vi "read single param.vi"(8 "error in (no error)":errorcluster, 10 "Parameter":string, 11 "PSP-603 in":refnum<class "PSP-603.lvclass">) -> (0 "error out":errorcluster, 2 "Data":string, 3 "PSP-603 out":refnum<class "PSP-603.lvclass">)   [LabVIEW 2025, in "Power Supply.lvlib" / "PSP-603.lvclass"]
uses:
  PSP-603.lvclass
  PSP-603.lvclass/PSP-603.ctl
panel:
  out "concatenated string":string
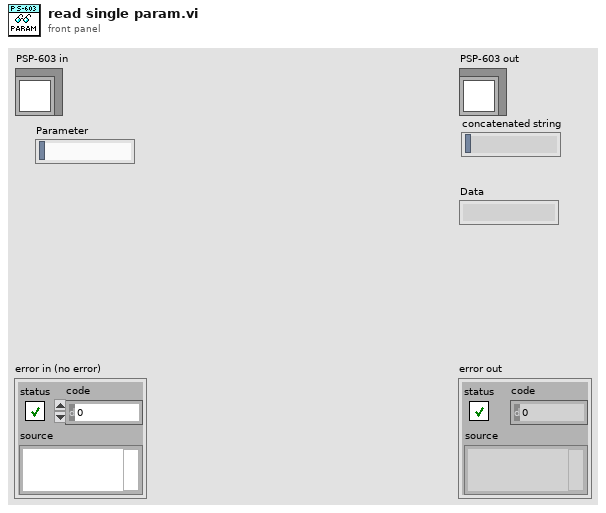
[diagram p1: front panel]
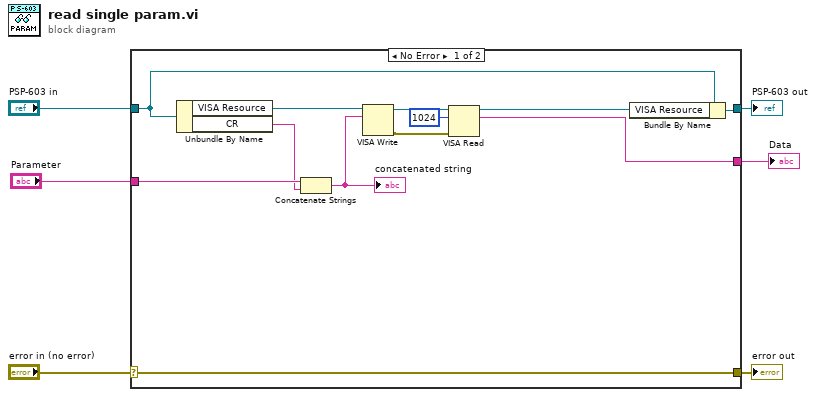
[diagram p0: block diagram]
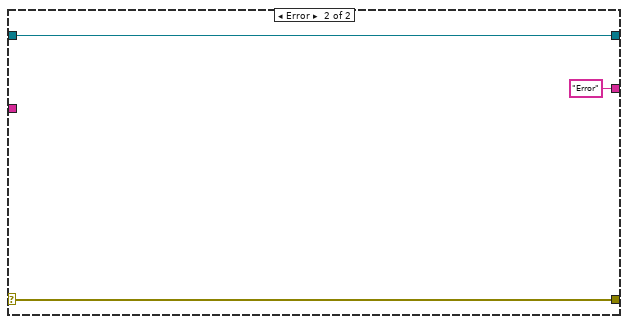
[diagram p2: hidden frame]
diagram:
  n1 = case shown="No Error" "error in (no error)" {
    selector: "error in (no error)" -> [w18 w21]
    tunnel: [w18 w21] -> w5
    tunnel: [w17 w20] -> w3
    tunnel: "PSP-603 in" -> [w16 w20]
    tunnel: "Parameter" -> [w10 _]
    tunnel: [w7 "Error" ("read buffer")] -> w1
    frame No Error {
      n2 = Unbundle By Name(w16) -> ("VISA Resource"=w15:refnum<visa-resource-name>, "CR"=w9:string)
      n3 = Concatenate Strings(w10, w9) -> (w8:string)
      "concatenated string" <- w8
      n4 = VISA Write(VISA resource name=w15, write buffer=w8) -> (VISA resource name out=w14:refnum<visa-resource-name>, error out=w13:errorcluster)  [unwired: 1 in, 1 out]
      n5 = VISA Read(VISA resource name=w14, byte count=u32 1024, error in (no error)=w13) -> (VISA resource name out=w11:refnum<visa-resource-name>, read buffer=w7:string)  [unwired: 2 out]
      n6 = Bundle By Name(cluster=w16, "VISA Resource"=w11) -> (w17:refnum<class "PSP-603.lvclass">)
    }
    frame Error {
    }
  }
  "error out" <- w5
  "PSP-603 out" <- w3
  "Data" <- w1
